vi "optz.vi"   [LabVIEW 2016, in "Moving Motor.lvrbt"]
uses:
  Moving Motor.lvrbt
  <vilib>/NXT/Block Support/NXT_InputPort.ctl
  <vilib>/NXT/Hardware/Plugins/Tetrix DC Motor/TetrixDCMotorAddress.ctl
  <vilib>/NXT/Dual Mode Library/Sensors/EV3_Color_Color.vi
  <vilib>/NXT/NXTIO Xnodes/NXTIONodeSubVIs/TETRIX IO Move DC Motors.vi
  <vilib>/NXT/NXTIO Xnodes/NXTIONodeSubVIs/TETRIX IO Stop DC Motors.vi
  <vilib>/NXT/Subs/LVHSConnector.ctl
  <vilib>/NXT/NXTIO Xnodes/AddressXNode/NXTIOAddress.xnode
  <vilib>/NXT/NXTIO Xnodes/NXTIOXNode/NXTIO.xnode
  <vilib>/NXT/LegoClasses/BrickReference/BrickReference.lvclass
types:
  T1 = typedef "NXT_InputPort.ctl" = u32
  T2 = typedef "LVHSConnector.ctl" = refnum<class "BrickReference.lvclass">
  T3 = typedef "ColorSensorColors.ctl" = enum16{"No Color", "Black", "Blue", "Green", "Yellow", "Red", "White", "Brown"}
  T4 = typedef "TetrixDCMotorAddress.ctl" = i32
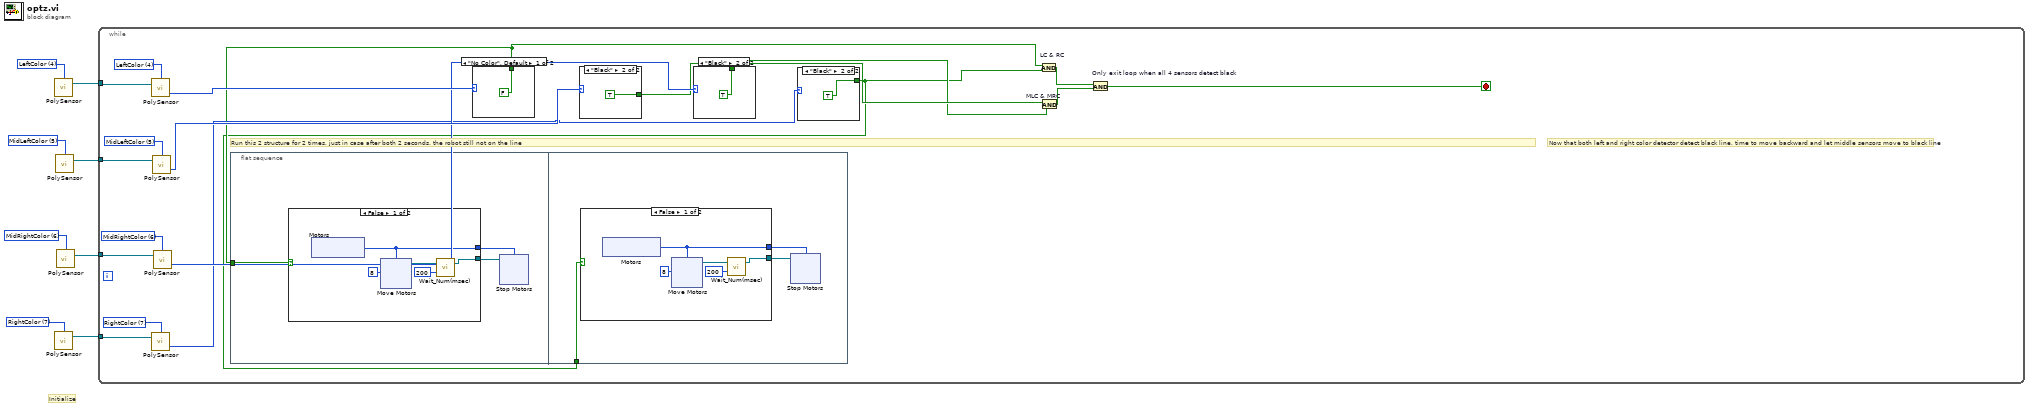
[diagram p0: block diagram]
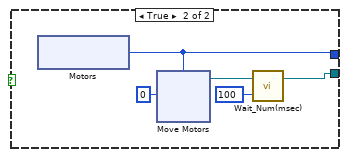
[diagram p2: hidden frame]
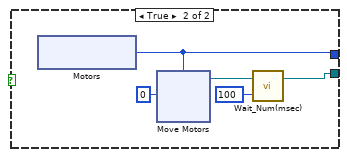
[diagram p3: hidden frame]
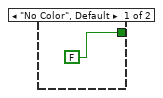
[diagram p4: hidden frame]
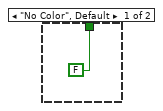
[diagram p5: hidden frame]
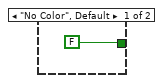
[diagram p6: hidden frame]
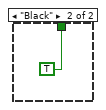
[diagram p7: hidden frame]
diagram:
  w5 = T1 6 items=["Port 1"=0, "Port 2"=1, "Port 3"=2, "Port 4"=3, "MidRightColor"=6] ("Port (Port 1)")
  w6 = T1 5 items=["Port 1"=0, "Port 2"=1, "Port 3"=2, "Port 4"=3, "MidLeftColor"=5] ("Port (Port 1)")
  w7 = T1 7 items=["Port 1"=0, "Port 2"=1, "Port 3"=2, "Port 4"=3, "LeftColor"=4, "RightColor"=7] ("Port (Port 1)")
  w8 = T1 4 items=["Port 1"=0, "Port 2"=1, "Port 3"=2, "Port 4"=3, "LeftColor"=4, "RightColor"=7] ("Port (Port 1)")
  # "Initialize"
  n1 = call-poly <vilib>:"PolySensor.vi"("Port (Port 1)"=w8) -> ("NXT/EV3"=w4:T2)  [unwired: 2 in, 1 out]
  n2 = call-poly <vilib>:"PolySensor.vi"("Port (Port 1)"=w7) -> ("NXT/EV3"=w1:T2)  [unwired: 2 in, 1 out]
  n3 = call-poly <vilib>:"PolySensor.vi"("Port (Port 1)"=w6) -> ("NXT/EV3"=w3:T2)  [unwired: 2 in, 1 out]
  n4 = call-poly <vilib>:"PolySensor.vi"("Port (Port 1)"=w5) -> ("NXT/EV3"=w2:T2)  [unwired: 2 in, 1 out]
  n5 = while {
    tunnel: w4 -> [w23]
    tunnel: w3 -> [w22]
    tunnel: w2 -> [w21]
    tunnel: w1 -> [w20]
    stop <- w11 stop-if-true
    w24 = T1 6 items=["Port 1"=0, "Port 2"=1, "Port 3"=2, "Port 4"=3, "MidRightColor"=6] ("Port (Port 1)")
    w25 = T1 5 items=["Port 1"=0, "Port 2"=1, "Port 3"=2, "Port 4"=3, "MidLeftColor"=5] ("Port (Port 1)")
    w26 = T1 7 items=["Port 1"=0, "Port 2"=1, "Port 3"=2, "Port 4"=3, "LeftColor"=4, "RightColor"=7] ("Port (Port 1)")
    w27 = T1 4 items=["Port 1"=0, "Port 2"=1, "Port 3"=2, "Port 4"=3, "LeftColor"=4, "RightColor"=7] ("Port (Port 1)")
    # "Run this 2 structure for 2 times, just in case after both 2 seconds, the robot still not on the line"
    # "Now that both left and right color detector detect black line, time to move backward and let middle sensors move to black line"
    n6 = call-poly <vilib>:"PolySensor.vi"("NXT/EV3"=w23, "Port (Port 1)"=w27) -> ("Detected Color"=w17:T3)  [unwired: 1 in, 1 out]
    n7 = call-poly <vilib>:"PolySensor.vi"("NXT/EV3"=w20, "Port (Port 1)"=w26) -> ("Detected Color"=w14:T3)  [unwired: 1 in, 1 out]
    n8 = call-poly <vilib>:"PolySensor.vi"("NXT/EV3"=w22, "Port (Port 1)"=w25) -> ("Detected Color"=w16:T3)  [unwired: 1 in, 1 out]
    n9 = call-poly <vilib>:"PolySensor.vi"("NXT/EV3"=w21, "Port (Port 1)"=w24) -> ("Detected Color"=w15:T3)  [unwired: 1 in, 1 out]
    n10 = flat-sequence {
      tunnel: w10 -> [w28]
      tunnel: w9 -> [w62]
      frame #0 {
        n11 = case shown="False" w28 {
          tunnel: [w37 w49] -> w30
          tunnel: [w36 w50] -> w29
          frame False {
            n12 = xnode "Motors"() -> ("Motor"=w36:T4)
            n13 = xnode "Move Motors"("Power/Speed 1"=i8 8, "Motors"=w36) -> ("NXT/EV3"=w39:T2)  [unwired: 1 in]
            n14 = call <vilib>:"Wait_Num(msec).vi"("Time (100 msec)"=u32 200, "NXT/EV3"=w39) -> ("NXT/EV3"=w37:T2)  [unwired: 2 in]
          }
          frame True {
            n15 = xnode "Motors"() -> ("Motor"=w50:T4)
            n16 = xnode "Move Motors"("Power/Speed 1"=i8 0, "Motors"=w50) -> ("NXT/EV3"=w52:T2)  [unwired: 1 in]
            n17 = call <vilib>:"Wait_Num(msec).vi"("Time (100 msec)"=u32 100, "NXT/EV3"=w52) -> ("NXT/EV3"=w49:T2)  [unwired: 2 in]
          }
        }
        n18 = xnode "Stop Motors"("Motors"=w29, "NXT/EV3"=w30) -> ()  [unwired: 1 out]
      }
      frame #1 {
        n19 = case shown="False" w62 {
          tunnel: [w71 w83] -> w64
          tunnel: [w70 w84] -> w63
          frame False {
            n20 = xnode "Motors"() -> ("Motor"=w70:T4)
            n21 = xnode "Move Motors"("Power/Speed 1"=i8 8, "Motors"=w70) -> ("NXT/EV3"=w73:T2)  [unwired: 1 in]
            n22 = call <vilib>:"Wait_Num(msec).vi"("Time (100 msec)"=u32 200, "NXT/EV3"=w73) -> ("NXT/EV3"=w71:T2)  [unwired: 2 in]
          }
          frame True {
            n23 = xnode "Motors"() -> ("Motor"=w84:T4)
            n24 = xnode "Move Motors"("Power/Speed 1"=i8 0, "Motors"=w84) -> ("NXT/EV3"=w86:T2)  [unwired: 1 in]
            n25 = call <vilib>:"Wait_Num(msec).vi"("Time (100 msec)"=u32 100, "NXT/EV3"=w86) -> ("NXT/EV3"=w83:T2)  [unwired: 2 in]
          }
        }
        n26 = xnode "Stop Motors"("Motors"=w63, "NXT/EV3"=w64) -> ()  [unwired: 1 out]
      }
    }
    n27 = case shown="\"No Color\", Default" w17 {
      tunnel: [FALSE TRUE] -> w10
      frame "No Color", Default {
      }
      frame "Black" {
      }
    }
    n28 = case shown="\"Black\"" w16 {
      tunnel: [FALSE TRUE] -> w13
      frame "No Color", Default {
      }
      frame "Black" {
      }
    }
    n29 = case shown="\"Black\"" w15 {
      tunnel: [FALSE TRUE] -> w12
      frame "No Color", Default {
      }
      frame "Black" {
      }
    }
    n30 = case shown="\"Black\"" w14 {
      tunnel: [FALSE TRUE] -> w9
      frame "No Color", Default {
      }
      frame "Black" {
      }
    }
    n31 = And "LC & RC"(x=w10, y=w9) -> (x .and. y?=w19:bool)
    n32 = And "MLC & MRC"(x=w13, y=w12) -> (x .and. y?=w18:bool)
    n33 = And "Only exit loop when all 4 sensors detect black"(x=w19, y=w18) -> (x .and. y?=w11:bool)
  }
